vi "ABB Norma 5000 Three Phase Measurement.vi"(7 "VT and CT Ratios":T1, 8 "error in (no error)":errorcluster, 11 "VISA session":refnum<visa-resource-name>) -> (0 "error out":errorcluster, 2 "Data":dbl[][](array[numeric]) format="%.2f", 3 "dup VISA session":refnum<visa-resource-name>)   [LabVIEW 2017]
doc: "This VI is an example that shows how to use the driver VIs. It configures the instrument and take a measurement. The following settings are configured with this VI:\n\n- Connection set to 3W\n- Config Input set all inputs to DC\n- Config Range set all phases to Autorange ON\n- Config Sync set phase to 1, Channel to voltage, Sync state to ON and Level to 25%\n- Averaging Interval set to 0.1 s\n- Initiate Continuous set state to ON\n- Averaging Status set timeout to 5 s \n- Measurements Functions set to U, I, P, S, Q and lambda on all three phases and total"
panel:
  # "L1                       L2                     L3                    Total"
  # "V"
  # "U"
  # "A"
  # "I"
  # "P"
  # "W"
  # "S"
  # "VA"
  # "Q"
  # "VAr"
  # "lambda"
  # "-"
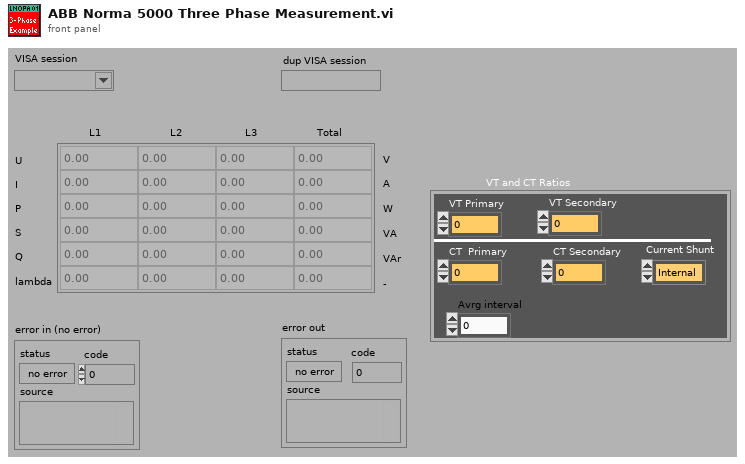
[diagram p1: front panel]
types:
  T1 = cluster{"VT Primary":dbl, "VT Secondary":dbl, "CT  Primary":dbl, "CT Secondary":dbl, "Current Shunt":enum16{"Internal", "External"}, "Avrg interval":dbl}
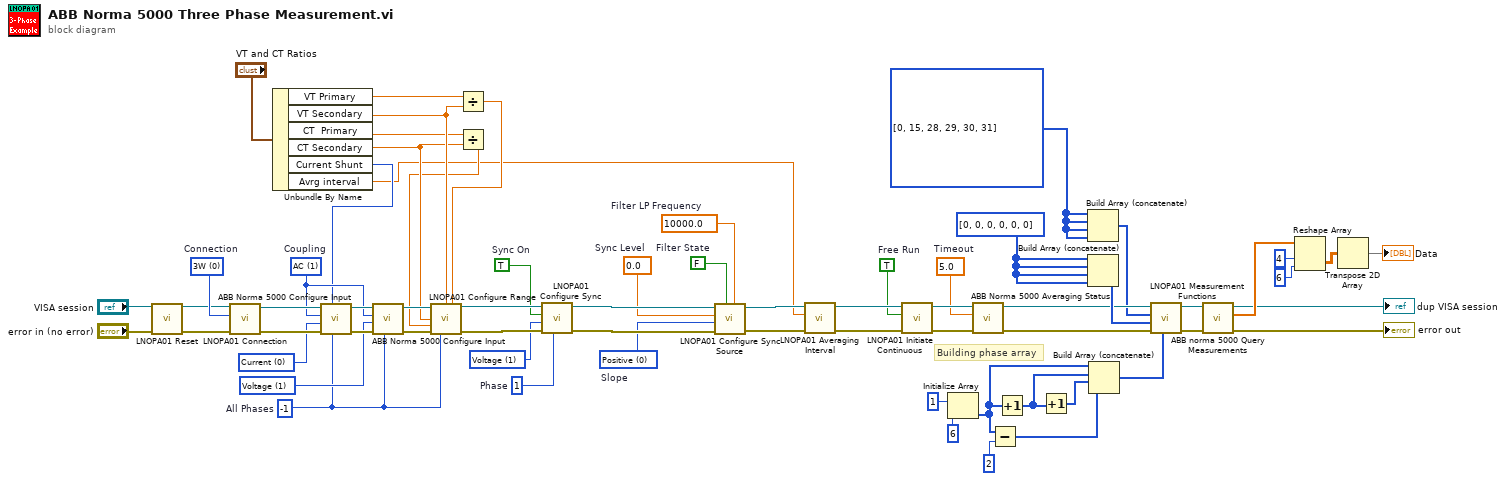
[diagram p0: block diagram]
diagram:
  w10 = i32[] [0, 15, 28, 29, 30, 31] items=["Voltage True RMS", "Voltage Mean", "Voltage Rectified Mean ", "Voltage Peak-To-Peak ", "Voltage Highest Value ", "Voltage Lowest Value ", "Voltage Crest Factor", "Voltage Absolute Phase", "Voltage True RMS Phase-To-Phase", "Voltage Harmonic", "Voltage TRMS Phase-To-Phase Harmonic", "Voltage Form Factor", "Voltage Harmonic Content", "Voltage Fundamental Content", "Voltage THD", "Current True RMS", "Current Mean", "Current Rectified Mean ", "Current Peak-To-Peak ", "Current Highest Value ", "Current Lowest Value", "Current Crest Factor", "Current Absolute Phase", "Current Harmonic", "Current Form Factor", "Current Harmonic Content", "Current Fundamental Content", "Current THD", "Power Active", "Power Apparent", "Power Reactive", "Power Factor", "Power Active Harmonic", "Power Apparent Harmonic", "Power Reactive Harmonic", "Power Factor Harmonic", "Power Corrected", "Phase", "Phase Harmonic", "Impedance", "Resistance Serial", "Resistance Parallel", "Reactance Serial", "Reactance Parallel", "Impedance Harmonic", "Resistance Serial Harmonic", "Resistance Parallel Harmonic", "Reactance Serial Harmonic", "Reactance Parallel Harmonic", "Frequency", "Averaging Interval", "Num of Avg Intervals Since Timer Reset", "Relative Time Since Timer Reset", "Shaft Torque", "Rotational Speed", "Mechanical Power", "Rotational Asynchronousity", "Motor Efficiency", "Raw Process Input Value "] ("Array Constant")
  w11 = 10000.0  # Filter LP Frequency
  w13 = 0 items=["Positive", "Negative"]  # Slope
  w12 = FALSE  # Filter State
  w28 = 1 items=["Current", "Voltage"] ("Channel")
  w29 = 0 items=["Current", "Voltage"] ("Channel")
  w16 = -1  # All Phases
  w27 = 1 items=["DC", "AC"]  # Coupling
  w15 = 1 items=["Current", "Voltage", "External"] ("Channel")
  w19 = 1  # Phase
  w21 = TRUE  # Sync On
  w14 = 0.0  # Sync Level
  w38 = 5.0  # Timeout
  w52 = TRUE  # Free Run
  w61 = i32[] [0, 0, 0, 0, 0, 0] items=["None", "Minimum", "Maximum", "Integral Positive", "Integral Negative", "Integral"] ("Modifier")
  w66 = 0 items=["3W", "2W"]  # Connection
  # "Building phase array"
  n1 = call "LNOPA01 Reset.vi"("VISA session"="VISA session", "error in (no error)"="error in (no error)") -> ("dup VISA session"=w33:refnum<visa-resource-name>, "error out"=w32:errorcluster)  [unwired: 12 in]
  n2 = call "LNOPA01 Connection.vi"("error in (no error)"=w32, "Connection"=w66, "VISA session"=w33) -> ("error out"=w64:errorcluster, "dup VISA session"=w65:refnum<visa-resource-name>)  [unwired: 6 in, 1 out]
  n3 = Unbundle By Name("VT and CT Ratios") -> ("VT Primary"=w8:dbl, "VT Secondary"=w7:dbl, "CT  Primary"=w6:dbl, "CT Secondary"=w5:dbl, "Current Shunt"=w2:enum16{"Internal", "External"}, "Avrg interval"=w1:dbl)
  n4 = call "ABB Norma 5000 Configure Input.vi"("Phase"=w16, "Current Shunt"=w2, "error in (no error)"=w64, "Channel"=w29, "Coupling"=w27, "VISA session"=w65) -> ("error out"=w30:errorcluster, "dup VISA session"=w31:refnum<visa-resource-name>)  [unwired: 4 in]
  n5 = call "ABB Norma 5000 Configure Input.vi"("Phase"=w16, "error in (no error)"=w30, "Channel"=w28, "Coupling"=w27, "VISA session"=w31) -> ("error out"=w26:errorcluster, "dup VISA session"=w25:refnum<visa-resource-name>)  [unwired: 5 in]
  n6 = Divide(x=w8, y=w7) -> (x/y=w4:dbl)
  n7 = Divide(x=w6, y=w5) -> (x/y=w3:dbl)
  n8 = call "LNOPA01 Configure Range.vi"("VISA session"=w25, "Voltage Range"=w7, "Voltage Scale Factor"=w4, "Current Range"=w5, "Current Scale Factor"=w3, "error in (no error)"=w26, "Phase"=w16) -> ("dup VISA session"=w24:refnum<visa-resource-name>, "error out"=w20:errorcluster)  [unwired: 7 in]
  n9 = call "LNOPA01 Configure Sync.vi"("Phase"=w19, "error in (no error)"=w20, "Channel"=w15, "State"=w21, "VISA session"=w24) -> ("error out"=w22:errorcluster, "dup VISA session"=w23:refnum<visa-resource-name>)  [unwired: 5 in]
  n10 = call "LNOPA01 Configure Sync Source.vi"("Filter LP Frequency"=w11, "Filter State"=w12, "error in (no error)"=w22, "Slope"=w13, "Level"=w14, "VISA session"=w23) -> ("error out"=w36:errorcluster, "dup VISA session"=w37:refnum<visa-resource-name>)  [unwired: 4 in]
  n11 = call "LNOPA01 Averaging Interval.vi"("error in (no error)"=w36, "Averaging Interval"=w1, "VISA session"=w37) -> ("error out"=w53:errorcluster, "dup VISA session"=w54:refnum<visa-resource-name>)  [unwired: 6 in, 1 out]
  n12 = call "LNOPA01 Initiate Continuous.vi"("error in (no error)"=w53, "State"=w52, "VISA session"=w54) -> ("error out"=w41:errorcluster, "dup VISA session"=w42:refnum<visa-resource-name>)  [unwired: 6 in, 1 out]
  n13 = Initialize Array(1 ("Element Data"), 6 ("Dimension Size")) -> (w49:i32[])
  n14 = call "ABB Norma 5000 Averaging Status.vi"("error in (no error)"=w41, "Timeout"=w38, "VISA session"=w42) -> ("error out"=w39:errorcluster, "dup VISA session"=w40:refnum<visa-resource-name>)  [unwired: 6 in, 1 out]
  n15 = Subtract(x=w49, y=2 ("Element Data")) -> (x-y=w56:i32[])
  n16 = Increment(x=w49) -> (x+1=w58:i32[])
  n17 = Increment(x=w58) -> (x+1=w57:i32[])
  n18 = Build Array (concatenate)(w10, w10, w10, w10) -> (w18:i32[])
  n19 = Build Array (concatenate)(w61, w61, w61, w61) -> (w60:i32[])
  n20 = Build Array (concatenate)(w49, w58, w57, w56) -> (w55:i32[])
  n21 = call "LNOPA01 Measurement Functions.vi"("Phase"=w55, "error in (no error)"=w39, "Modifier"=w60, "Measurement"=w18, "VISA session"=w40) -> ("error out"=w50:errorcluster, "dup VISA session"=w51:refnum<visa-resource-name>)  [unwired: 2 in, 3 out]
  n22 = call "ABB norma 5000 Query Measurements.vi"("error in (no error)"=w50, "VISA session"=w51) -> ("error out"=→"error out":errorcluster, "Data"=w48:dbl[], "dup VISA session"=→"dup VISA session":refnum<visa-resource-name>)  [unwired: 7 in]
  n23 = Reshape Array(w48, 4 ("Dimension Size"), 6 ("Dimension Size")) -> (w45:dbl[][])
  n24 = Transpose 2D Array(2D array=w45) -> (transposed array=→"Data":dbl[][])
